vi "EQUIPMENT_MANAGER.vi"() -> ()   [LabVIEW 2018]
panel:
  in  "MAIN_MINIMIZE":bool
  out "MAIN_STATUS_TRANS":bool caption="CAUTION!"
  out "MAIN_INFO_USER":string
  in  "MAIN_CLOSE":bool
  out "MAIN_INFO_NOTE":string caption="String"
  in  "MAIN_TAB":enum32{"DASHBOARD", "REGISTER", "SHIPPING"}(tab)
  in  "reg_PRINT BUTTON":bool caption="Button"
  out "VALIDATED":bool
  in  "reg_DELETE BUTTON":bool
  in  "VALIDATE BUTTON":bool
  in  "FIND BUTTON":bool
  in  "DOWNLOAD BUTTON":bool
  in  "reg_UPLOAD BUTTON":bool
  out "IMAGE":picture
  in  "REGISTER BUTTON":bool
  in  "MODEL   :":string
  in  "DUE DATE:":timestamp format="%<%d-%b-%Y>T"
  in  "STATUS  :":T1(ring)
  in  "MANF.   :":string
  in  "SN      :":string
  in  "PN      :":string
  in  "DESC.   :":string
  in  "AREA    :":string
  in  "REGISTRATION NUMBER":string caption="REG. NO.:"
  in  "REGISTER TABLE":i32(listbox)
  in  "REMARKS  :":string
  in  "UPLOAD BUTTON":bool
  in  "PRINT BUTTON":bool
  in  "DELETE BUTTON":bool
  in  "TO       :":string
  in  "DATE     :":timestamp format="%<%d-%b-%Y>T"
  in  "NO. SP.  :":string
  in  "SHIPPING TABLE":i32(listbox)
  in  "PACKED BY:":string
  in  "SENT BY  :":string
  in  "SP IN/OUT":enum32{"Item 0", "Item 1"}(radio)
  in  "ADD BUTTON":bool
  in  "REG. NO. :":string
  # "EQUIPMENT MANAGER"
  # "(unit)"
  # "(person)"
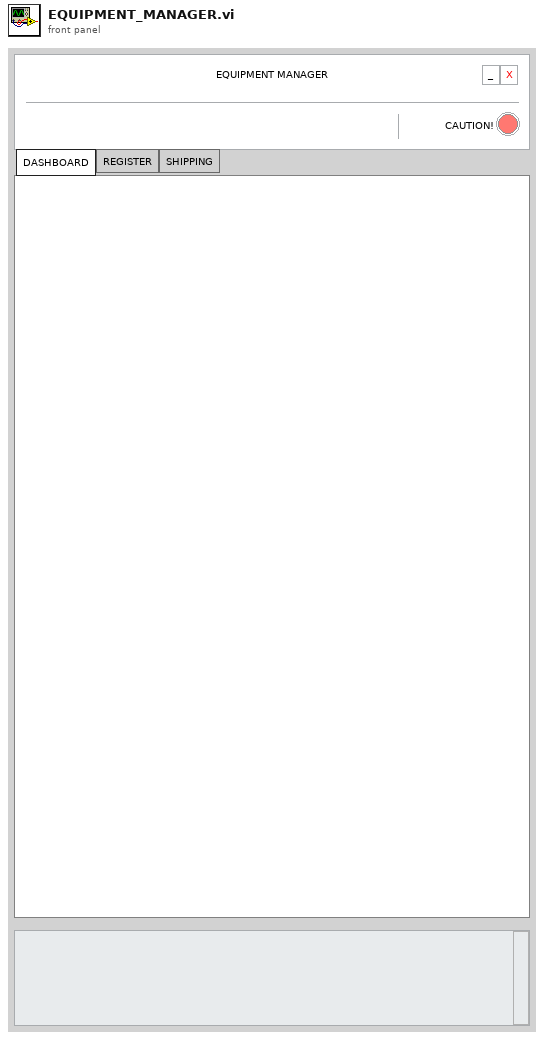
[diagram p1: front panel]
types:
  T1 = enum16{"SERVICABLE", "CALIBRATION", "REPAIR", "RESERVED", "USED", "SCRAP"}
  T2 = enum32{"Size Tabs To Contents", "Size All Tabs to Largest Tab", "Fixed Tab Size"}
  T3 = enum32{"Invalid", "Standard", "Closed", "Hidden", "Minimized", "Maximized"}
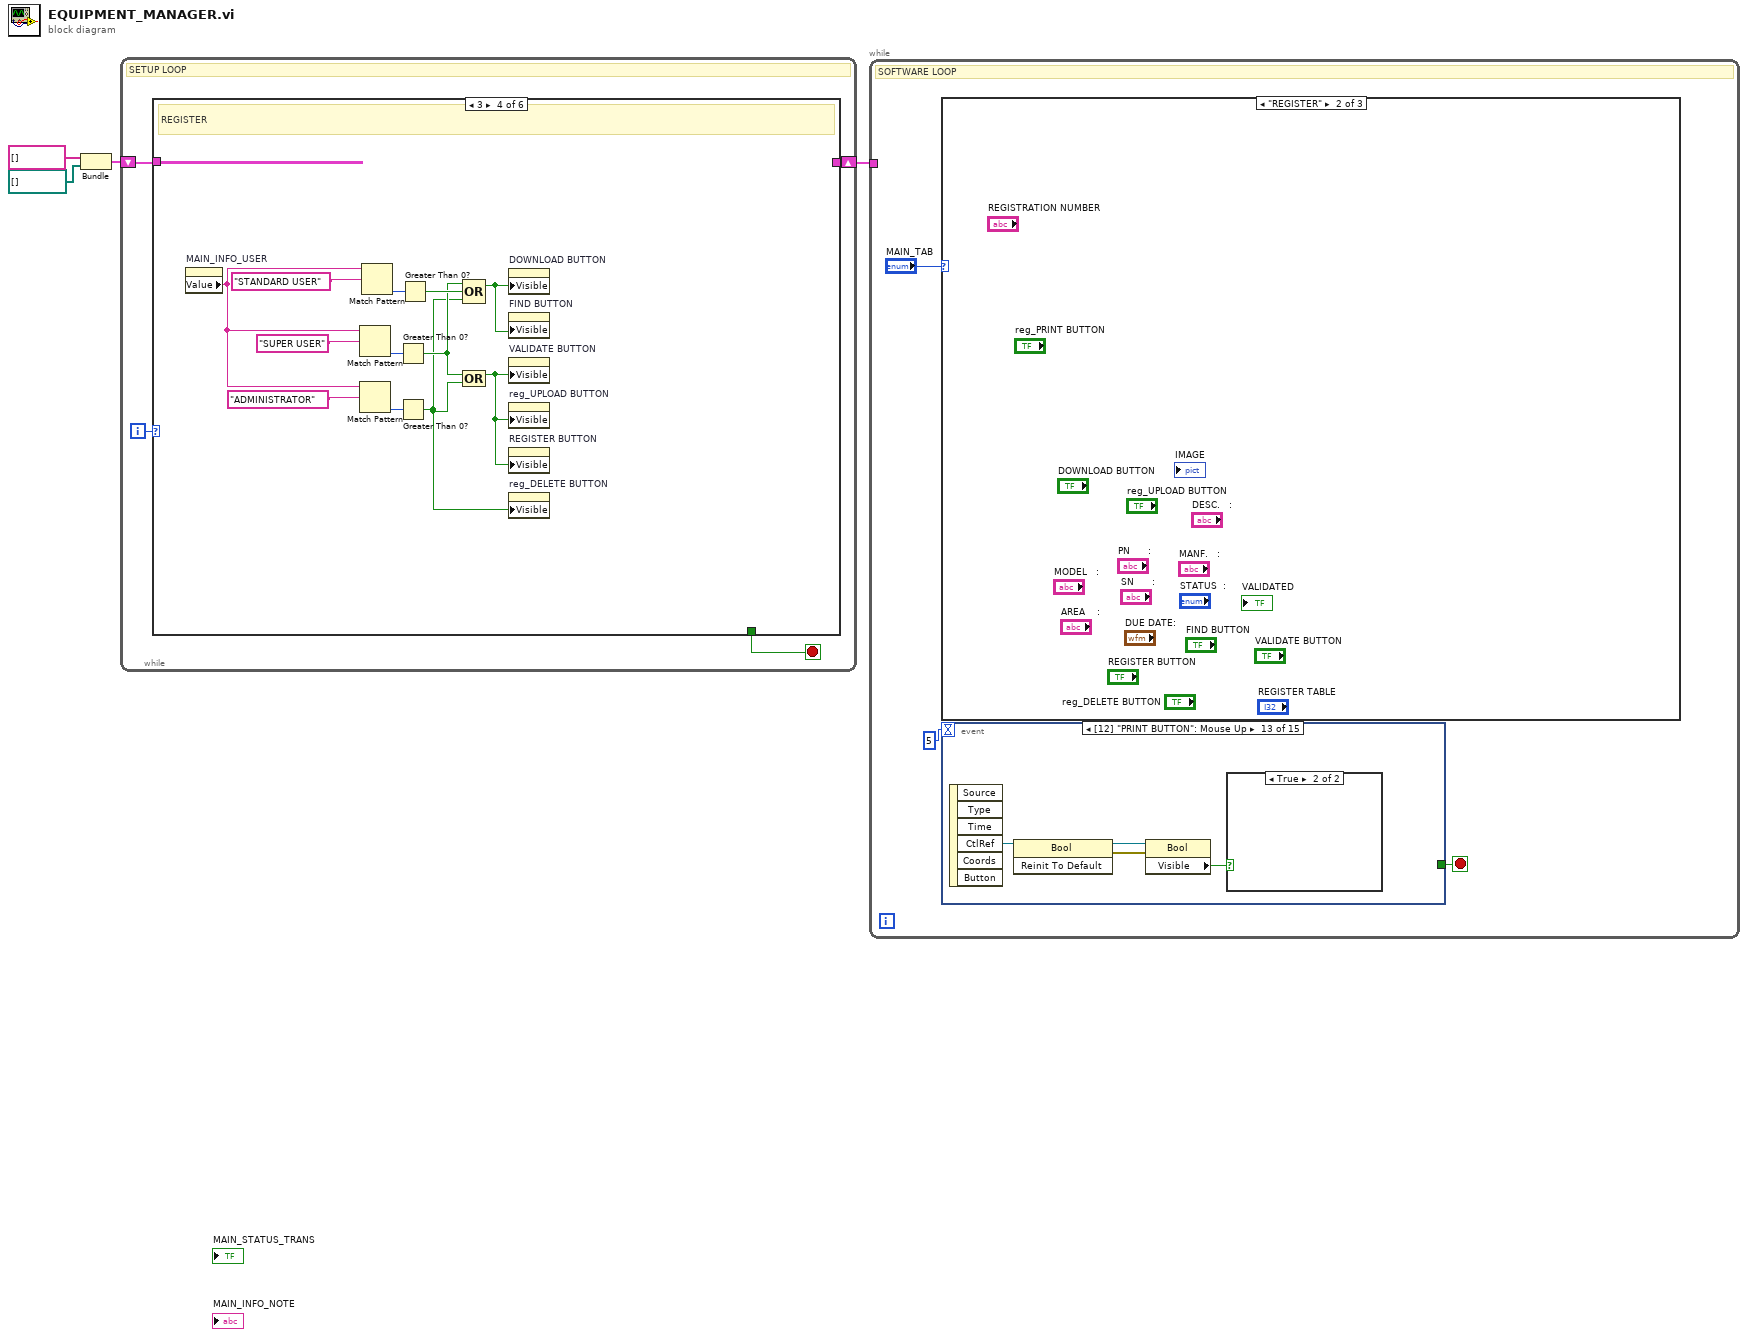
[diagram p0: block diagram]
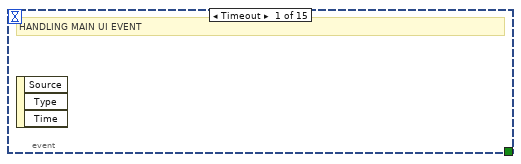
[diagram p2: hidden frame]
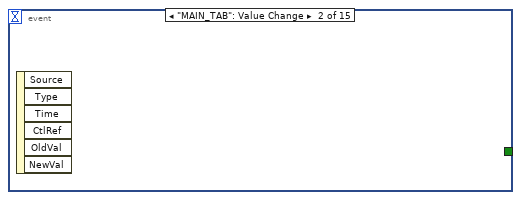
[diagram p3: hidden frame]
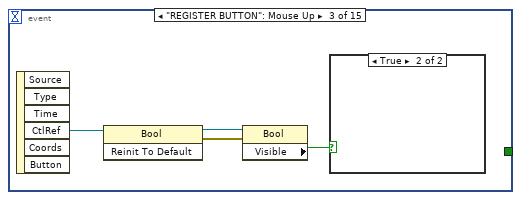
[diagram p4: hidden frame]
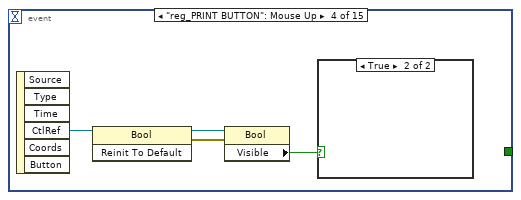
[diagram p6: hidden frame]
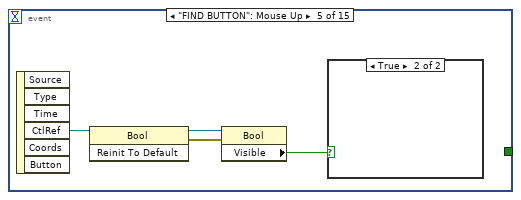
[diagram p8: hidden frame]
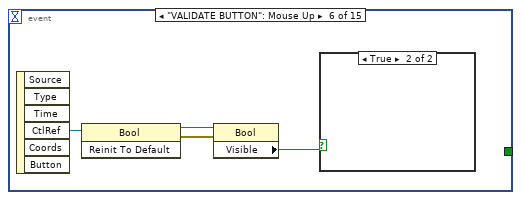
[diagram p10: hidden frame]
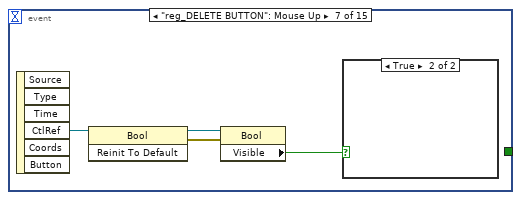
[diagram p12: hidden frame]
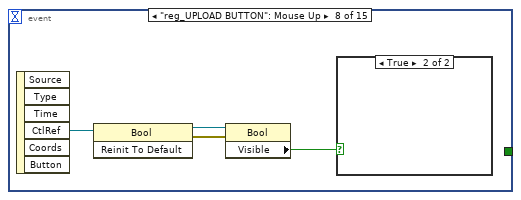
[diagram p14: hidden frame]
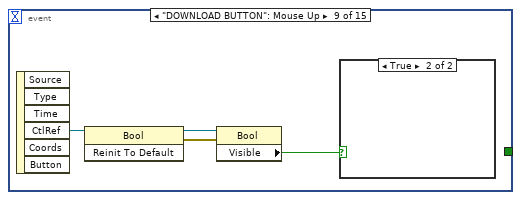
[diagram p16: hidden frame]
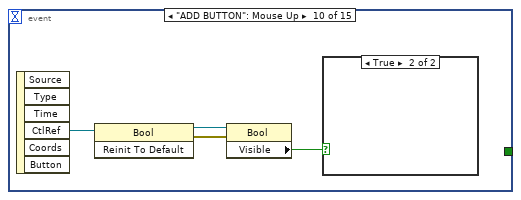
[diagram p18: hidden frame]
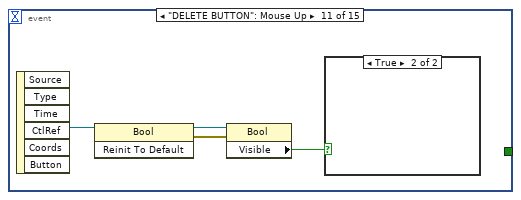
[diagram p20: hidden frame]
diagram:
  n1 = Bundle(string[] [], path[] []) -> (w1:cluster{string[], path[]})  [unwired: 1 in]
  n2 = while {
    shift-right: [w7] -> w2
    shift-left: w1 -> [w6]
    i -> [w8]
    stop <- w5 stop-if-true
    # "SETUP LOOP"
    n3 = case shown="3" w8 {
      tunnel: w6 -> [w9 w12 _ _ _ _]
      tunnel: [w9 w12 _ _ _ _] -> w7
      tunnel: [_ _ _ _ _ TRUE] -> w5
      frame 0, Default {
        # "SEQ #0\nCOMMAND LINE ARGUMENTS"
      }
      frame 1 {
        # "SEQ #1\nINIT ALL TERMINAL; DISPLAY USER INFO; ADJUST UNIFORM TAB SIZE"
        n4 = control-ref of="This VI"() -> (w13:refnum<vi>)
        n5 = invoke class="VI" method="Default Vals.Reinit All"(reference=w13) -> (error out=w11:errorcluster)  [unwired: 2 in, 2 out]
        n6 = property on="MAIN_TAB" class="TabCtl (strict)"(error in=w11, "TabSize"=T2."Size All Tabs to Largest Tab" ("Tab Size")) -> ()  [unwired: 1 in, 2 out]
      }
      frame 2 {
        # "DASHBOARD"
        "MAIN_INFO_USER" <- "ADMINISTRATOR" ("MAIN_INFO_USER")
      }
      frame 3 {
        # "REGISTER"
        n7 = property on="MAIN_INFO_USER" class="Str"() -> ("Value"=w20:string)  [unwired: 2 in, 2 out]
        n8 = Match Pattern(string=w20, regular expression="SUPER USER") -> (offset past match=w25:i32)  [unwired: 1 in, 3 out]
        n9 = Match Pattern(string=w20, regular expression="ADMINISTRATOR") -> (offset past match=w21:i32)  [unwired: 1 in, 3 out]
        n10 = Match Pattern(string=w20, regular expression="STANDARD USER") -> (offset past match=w23:i32)  [unwired: 1 in, 3 out]
        n11 = Greater Than 0?(x=w25) -> (x > 0?=w18:bool)
        n12 = Greater Than 0?(x=w21) -> (x > 0?=w16:bool)
        n13 = Greater Than 0?(x=w23) -> (x > 0?=w19:bool)
        n14 = Compound Arithmetic op=OR(w18, w19, w16) -> (w17:bool)
        n15 = Compound Arithmetic op=OR(w18, w16) -> (w15:bool)
        n16 = property on="DOWNLOAD BUTTON" class="Bool"("Visible"=w17) -> ()  [unwired: 2 in, 2 out]
        n17 = property on="FIND BUTTON" class="Bool"("Visible"=w17) -> ()  [unwired: 2 in, 2 out]
        n18 = property on="VALIDATE BUTTON" class="Bool"("Visible"=w15) -> ()  [unwired: 2 in, 2 out]
        n19 = property on="reg_UPLOAD BUTTON" class="Bool"("Visible"=w15) -> ()  [unwired: 2 in, 2 out]
        n20 = property on="REGISTER BUTTON" class="Bool"("Visible"=w15) -> ()  [unwired: 2 in, 2 out]
        n21 = property on="reg_DELETE BUTTON" class="Bool"("Visible"=w16) -> ()  [unwired: 2 in, 2 out]
      }
      frame 4 {
        # "SHIPPING"
        n22 = property on="MAIN_INFO_USER" class="Str"() -> ("Value"=w32:string)  [unwired: 2 in, 2 out]
        n23 = Match Pattern(string=w32, regular expression="SUPER USER") -> (offset past match=w31:i32)  [unwired: 1 in, 3 out]
        n24 = Match Pattern(string=w32, regular expression="ADMINISTRATOR") -> (offset past match=w30:i32)  [unwired: 1 in, 3 out]
        n25 = Greater Than 0?(x=w31) -> (x > 0?=w29:bool)
        n26 = Greater Than 0?(x=w30) -> (x > 0?=w28:bool)
        n27 = Compound Arithmetic op=OR(w29, w28) -> (w27:bool)
        n28 = property on="ADD BUTTON" class="Bool"("Visible"=w27) -> ()  [unwired: 2 in, 2 out]
        n29 = property on="UPLOAD BUTTON" class="Bool"("Visible"=w27) -> ()  [unwired: 2 in, 2 out]
        n30 = property on="PRINT BUTTON" class="Bool"("Visible"=w27) -> ()  [unwired: 2 in, 2 out]
        n31 = property on="DELETE BUTTON" class="Bool"("Visible"=w27) -> ()  [unwired: 2 in, 2 out]
      }
      frame 5 {
        # "FINALIZE"
      }
    }
  }
  n32 = while {
    tunnel: w2 -> [_]
    stop <- w36 stop-if-true
    # "SOFTWARE LOOP"
    n33 = case shown="\"REGISTER\"" "MAIN_TAB" {
      frame "DASHBOARD", Default {
      }
      frame "REGISTER" {
      }
      frame "SHIPPING" {
      }
    }
    n34 = event shown="[12] \"PRINT BUTTON\": Mouse Up" {
      selector: _ -> [_ _ _ _ _ _ _ _ _ _ _ _ _ _ _]
      dyn-events: _ -> [_ _ _ _ _ _ _ _ _ _ _ _ _ _ _]
      timeout: 5 -> [_ _ _ _ _ _ _ _ _ _ _ _ _ _ _]
      tunnel: [_ _ _ _ _ _ _ _ _ _ _ _ _ _ TRUE] -> w36
      event Timeout {
        # "HANDLING MAIN UI EVENT"
        n35 = event-data() -> ()  [unwired: 1 in, 3 out]
      }
      event "MAIN_TAB": Value Change {
        n36 = event-data() -> ()  [unwired: 1 in, 6 out]
      }
      event "REGISTER BUTTON": Mouse Up {
        n37 = event-data() -> ("CtlRef"=w42:refnum<vi>)  [unwired: 1 in, 5 out]
        n38 = invoke class="Bool" method="Reinit To Default"(reference=w42) -> (reference out=w41:refnum<vi>, error out=w40:errorcluster)  [unwired: 2 in, 1 out]
        n39 = property class="Bool"(reference=w41, error in=w40) -> ("Visible"=w39:bool)  [unwired: 2 out]
        n40 = case shown="True" w39 {
          frame False {
          }
          frame True {
          }
        }
      }
      event "reg_PRINT BUTTON": Mouse Up {
        n41 = event-data() -> ("CtlRef"=w46:refnum<vi>)  [unwired: 1 in, 5 out]
        n42 = invoke class="Bool" method="Reinit To Default"(reference=w46) -> (reference out=w45:refnum<vi>, error out=w44:errorcluster)  [unwired: 2 in, 1 out]
        n43 = property class="Bool"(reference=w45, error in=w44) -> ("Visible"=w43:bool)  [unwired: 2 out]
        n44 = case shown="True" w43 {
          frame False {
          }
          frame True {
          }
        }
      }
      event "FIND BUTTON": Mouse Up {
        n45 = event-data() -> ("CtlRef"=w48:refnum<vi>)  [unwired: 1 in, 5 out]
        n46 = invoke class="Bool" method="Reinit To Default"(reference=w48) -> (reference out=w50:refnum<vi>, error out=w49:errorcluster)  [unwired: 2 in, 1 out]
        n47 = property class="Bool"(reference=w50, error in=w49) -> ("Visible"=w47:bool)  [unwired: 2 out]
        n48 = case shown="True" w47 {
          frame False {
          }
          frame True {
          }
        }
      }
      event "VALIDATE BUTTON": Mouse Up {
        n49 = event-data() -> ("CtlRef"=w52:refnum<vi>)  [unwired: 1 in, 5 out]
        n50 = invoke class="Bool" method="Reinit To Default"(reference=w52) -> (reference out=w54:refnum<vi>, error out=w53:errorcluster)  [unwired: 2 in, 1 out]
        n51 = property class="Bool"(reference=w54, error in=w53) -> ("Visible"=w51:bool)  [unwired: 2 out]
        n52 = case shown="True" w51 {
          frame False {
          }
          frame True {
          }
        }
      }
      event "reg_DELETE BUTTON": Mouse Up {
        n53 = event-data() -> ("CtlRef"=w56:refnum<vi>)  [unwired: 1 in, 5 out]
        n54 = invoke class="Bool" method="Reinit To Default"(reference=w56) -> (reference out=w58:refnum<vi>, error out=w57:errorcluster)  [unwired: 2 in, 1 out]
        n55 = property class="Bool"(reference=w58, error in=w57) -> ("Visible"=w55:bool)  [unwired: 2 out]
        n56 = case shown="True" w55 {
          frame False {
          }
          frame True {
          }
        }
      }
      event "reg_UPLOAD BUTTON": Mouse Up {
        n57 = event-data() -> ("CtlRef"=w60:refnum<vi>)  [unwired: 1 in, 5 out]
        n58 = invoke class="Bool" method="Reinit To Default"(reference=w60) -> (reference out=w62:refnum<vi>, error out=w61:errorcluster)  [unwired: 2 in, 1 out]
        n59 = property class="Bool"(reference=w62, error in=w61) -> ("Visible"=w59:bool)  [unwired: 2 out]
        n60 = case shown="True" w59 {
          frame False {
          }
          frame True {
          }
        }
      }
      event "DOWNLOAD BUTTON": Mouse Up {
        n61 = event-data() -> ("CtlRef"=w64:refnum<vi>)  [unwired: 1 in, 5 out]
        n62 = invoke class="Bool" method="Reinit To Default"(reference=w64) -> (reference out=w66:refnum<vi>, error out=w65:errorcluster)  [unwired: 2 in, 1 out]
        n63 = property class="Bool"(reference=w66, error in=w65) -> ("Visible"=w63:bool)  [unwired: 2 out]
        n64 = case shown="True" w63 {
          frame False {
          }
          frame True {
          }
        }
      }
      event "ADD BUTTON": Mouse Up {
        n65 = event-data() -> ("CtlRef"=w68:refnum<vi>)  [unwired: 1 in, 5 out]
        n66 = invoke class="Bool" method="Reinit To Default"(reference=w68) -> (reference out=w70:refnum<vi>, error out=w69:errorcluster)  [unwired: 2 in, 1 out]
        n67 = property class="Bool"(reference=w70, error in=w69) -> ("Visible"=w67:bool)  [unwired: 2 out]
        n68 = case shown="True" w67 {
          frame False {
          }
          frame True {
          }
        }
      }
      event "DELETE BUTTON": Mouse Up {
        n69 = event-data() -> ("CtlRef"=w72:refnum<vi>)  [unwired: 1 in, 5 out]
        n70 = invoke class="Bool" method="Reinit To Default"(reference=w72) -> (reference out=w74:refnum<vi>, error out=w73:errorcluster)  [unwired: 2 in, 1 out]
        n71 = property class="Bool"(reference=w74, error in=w73) -> ("Visible"=w71:bool)  [unwired: 2 out]
        n72 = case shown="True" w71 {
          frame False {
          }
          frame True {
          }
        }
      }
      event "UPLOAD BUTTON": Mouse Up {
        n73 = event-data() -> ("CtlRef"=w76:refnum<vi>)  [unwired: 1 in, 5 out]
        n74 = invoke class="Bool" method="Reinit To Default"(reference=w76) -> (reference out=w78:refnum<vi>, error out=w77:errorcluster)  [unwired: 2 in, 1 out]
        n75 = property class="Bool"(reference=w78, error in=w77) -> ("Visible"=w75:bool)  [unwired: 2 out]
        n76 = case shown="True" w75 {
          frame False {
          }
          frame True {
          }
        }
      }
      event "PRINT BUTTON": Mouse Up {
        n77 = event-data() -> ("CtlRef"=w80:refnum<vi>)  [unwired: 1 in, 5 out]
        n78 = invoke class="Bool" method="Reinit To Default"(reference=w80) -> (reference out=w82:refnum<vi>, error out=w81:errorcluster)  [unwired: 2 in, 1 out]
        n79 = property class="Bool"(reference=w82, error in=w81) -> ("Visible"=w79:bool)  [unwired: 2 out]
        n80 = case shown="True" w79 {
          frame False {
          }
          frame True {
          }
        }
      }
      event "MAIN_MINIMIZE": Mouse Up {
        n81 = event-data() -> ("CtlRef"=w84:refnum<vi>)  [unwired: 1 in, 5 out]
        n82 = invoke class="Bool" method="Reinit To Default"(reference=w84) -> (error out=w83:errorcluster)  [unwired: 2 in, 2 out]
        n83 = control-ref of="This VI"() -> (w86:refnum<vi>)
        n84 = property class="VI"(reference=w86, error in=w83, "FP.State"=T3."Minimized" ("Front Panel Window:State")) -> ()  [unwired: 2 out]
      }
      event "MAIN_CLOSE": Mouse Up {
        n85 = event-data() -> ("CtlRef"=w88:refnum<vi>)  [unwired: 1 in, 3 out]
        n86 = invoke class="Bool" method="Reinit To Default"(reference=w88) -> ()  [unwired: 2 in, 3 out]
      }
    }
  }
